vi "MFC_LED_training.vi"() -> ()   [LabVIEW 2021]
uses:
  OdorSensorArray/labview 2016 code/osa_global_save2.vi
  <vilib>/measure/NI_MABase.lvlib
panel:
  in  "Max Voltage 3":dbl=4.5 min=0.0 max=5.0 step=0.1 format="%.2f"
  in  "Min Voltage 3":dbl=0.5 min=0.0 max=5.0 step=0.1 format="%.2f"
  in  "Frequency (Hz) burst":dbl=1.0 step=0.1 format="%.3f"
  in  "Phase_delay":dbl=1.0 step=0.1 format="%.3f"
  in  "Duty cycle (%) 2":dbl=1.0 step=0.1 format="%.3f"
  in  "Function 2":u16(ring) items=["Sine Wave", "Triangle Wave", "Square Wave", "Sawtooth Wave"]
  out "Waveform Chart 2":dbl(graph)
  in  "Duty cycle (%)":dbl=1.0 step=0.1 format="%.3f"
  out "Error U3-2 A0":string
  out "PID / flow":cluster{"Value Read":dbl, "Value Read":dbl}(graph)
  in  "Dilusion_lj2_DAC1":dbl step=0.1 format="%.4f"
  out "Error  PID_Save":string
  out "error write":errorcluster
  in  "Save file":bool
  in  "save data folder":path
  out "appended path":path
  out "AIN0: PID":dbl format="%.6f"
  out "MFC I/O":cluster{"Value Read":dbl, "Value Read":dbl}(graph)
  out "AIN2: MFCr":dbl format="%.6f"
  out "AIN1: MFCw":dbl format="%.6f"
  out "Waveform Chart":dbl(graph)
  out "Error DAC1,B":string
  out "error read":errorcluster
  in  "Background_DAC1":dbl step=0.1 format="%.4f"
  in  "Update Interval (ms)":u32=20
  out "Error_DAC0":string
  in  "Function":u16(ring) items=["Sine Wave", "Triangle Wave", "Square Wave", "Sawtooth Wave"]
  in  "Min Voltage":dbl=0.5 min=0.0 max=5.0 step=0.1 format="%.2f"
  in  "Max Voltage":dbl=4.5 min=0.0 max=5.0 step=0.1 format="%.2f"
  in  "Frequency (Hz)":dbl=1.0 step=0.1 format="%.3f"
  in  "Stop":bool
  # "Updates DAC0 at the specified update interval in order to build time series waveforms.  The\nupdate interval is set to 20 ms by default, but can be set lower based on the execution times\ndiscussed in Section 3.1 of the U3 User's Guide.  Uses the first found U3.\n\nWith a software timed application such as this, you might be able to reduce timing jitter (caused\nby the operating system) by increasing the priority of this process (labview.exe) in Windows\nTask Manager."
  # "MFC"
  # "LED"
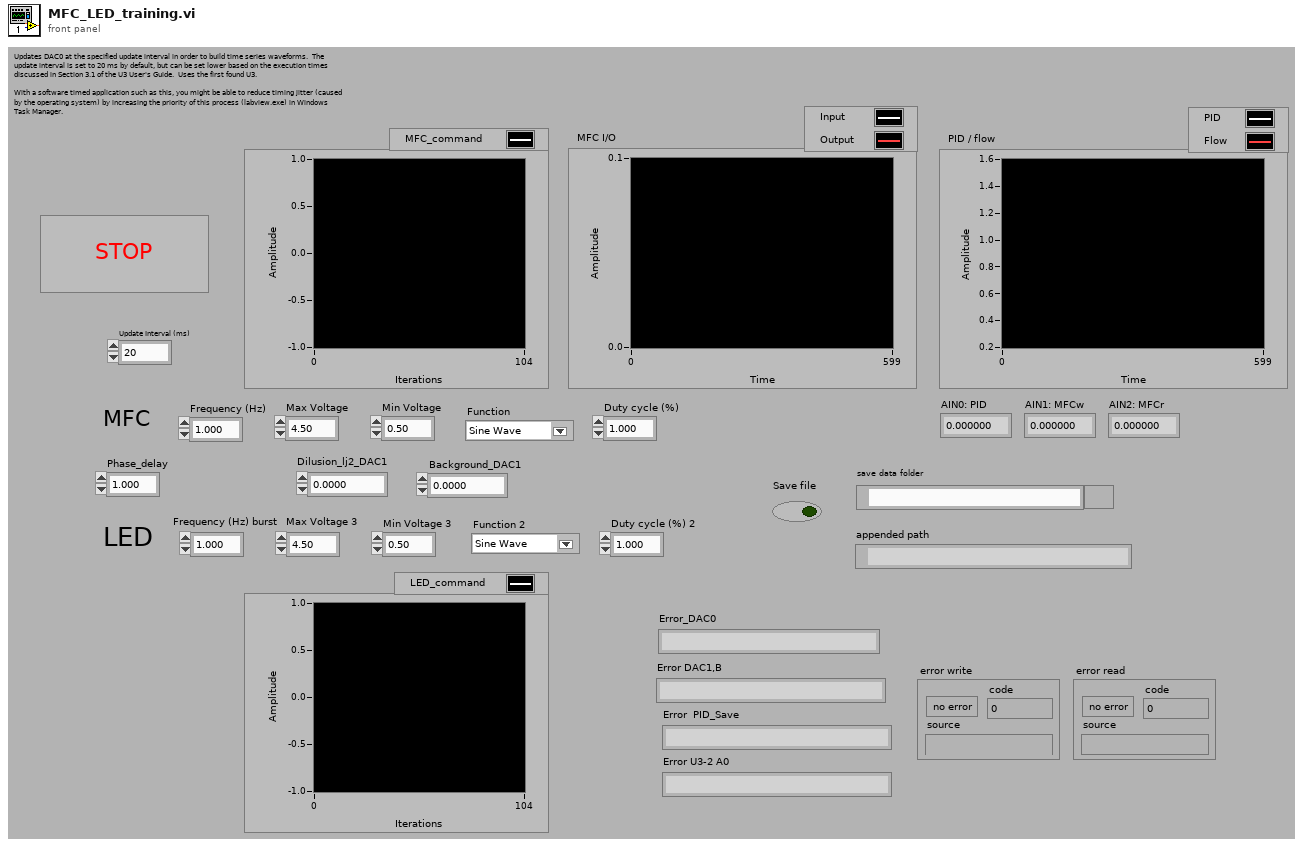
[diagram p1: front panel]
types:
  T1 = enum16{"open", "replace", "create", "open or create", "replace or create", "replace or create with confirmation"}
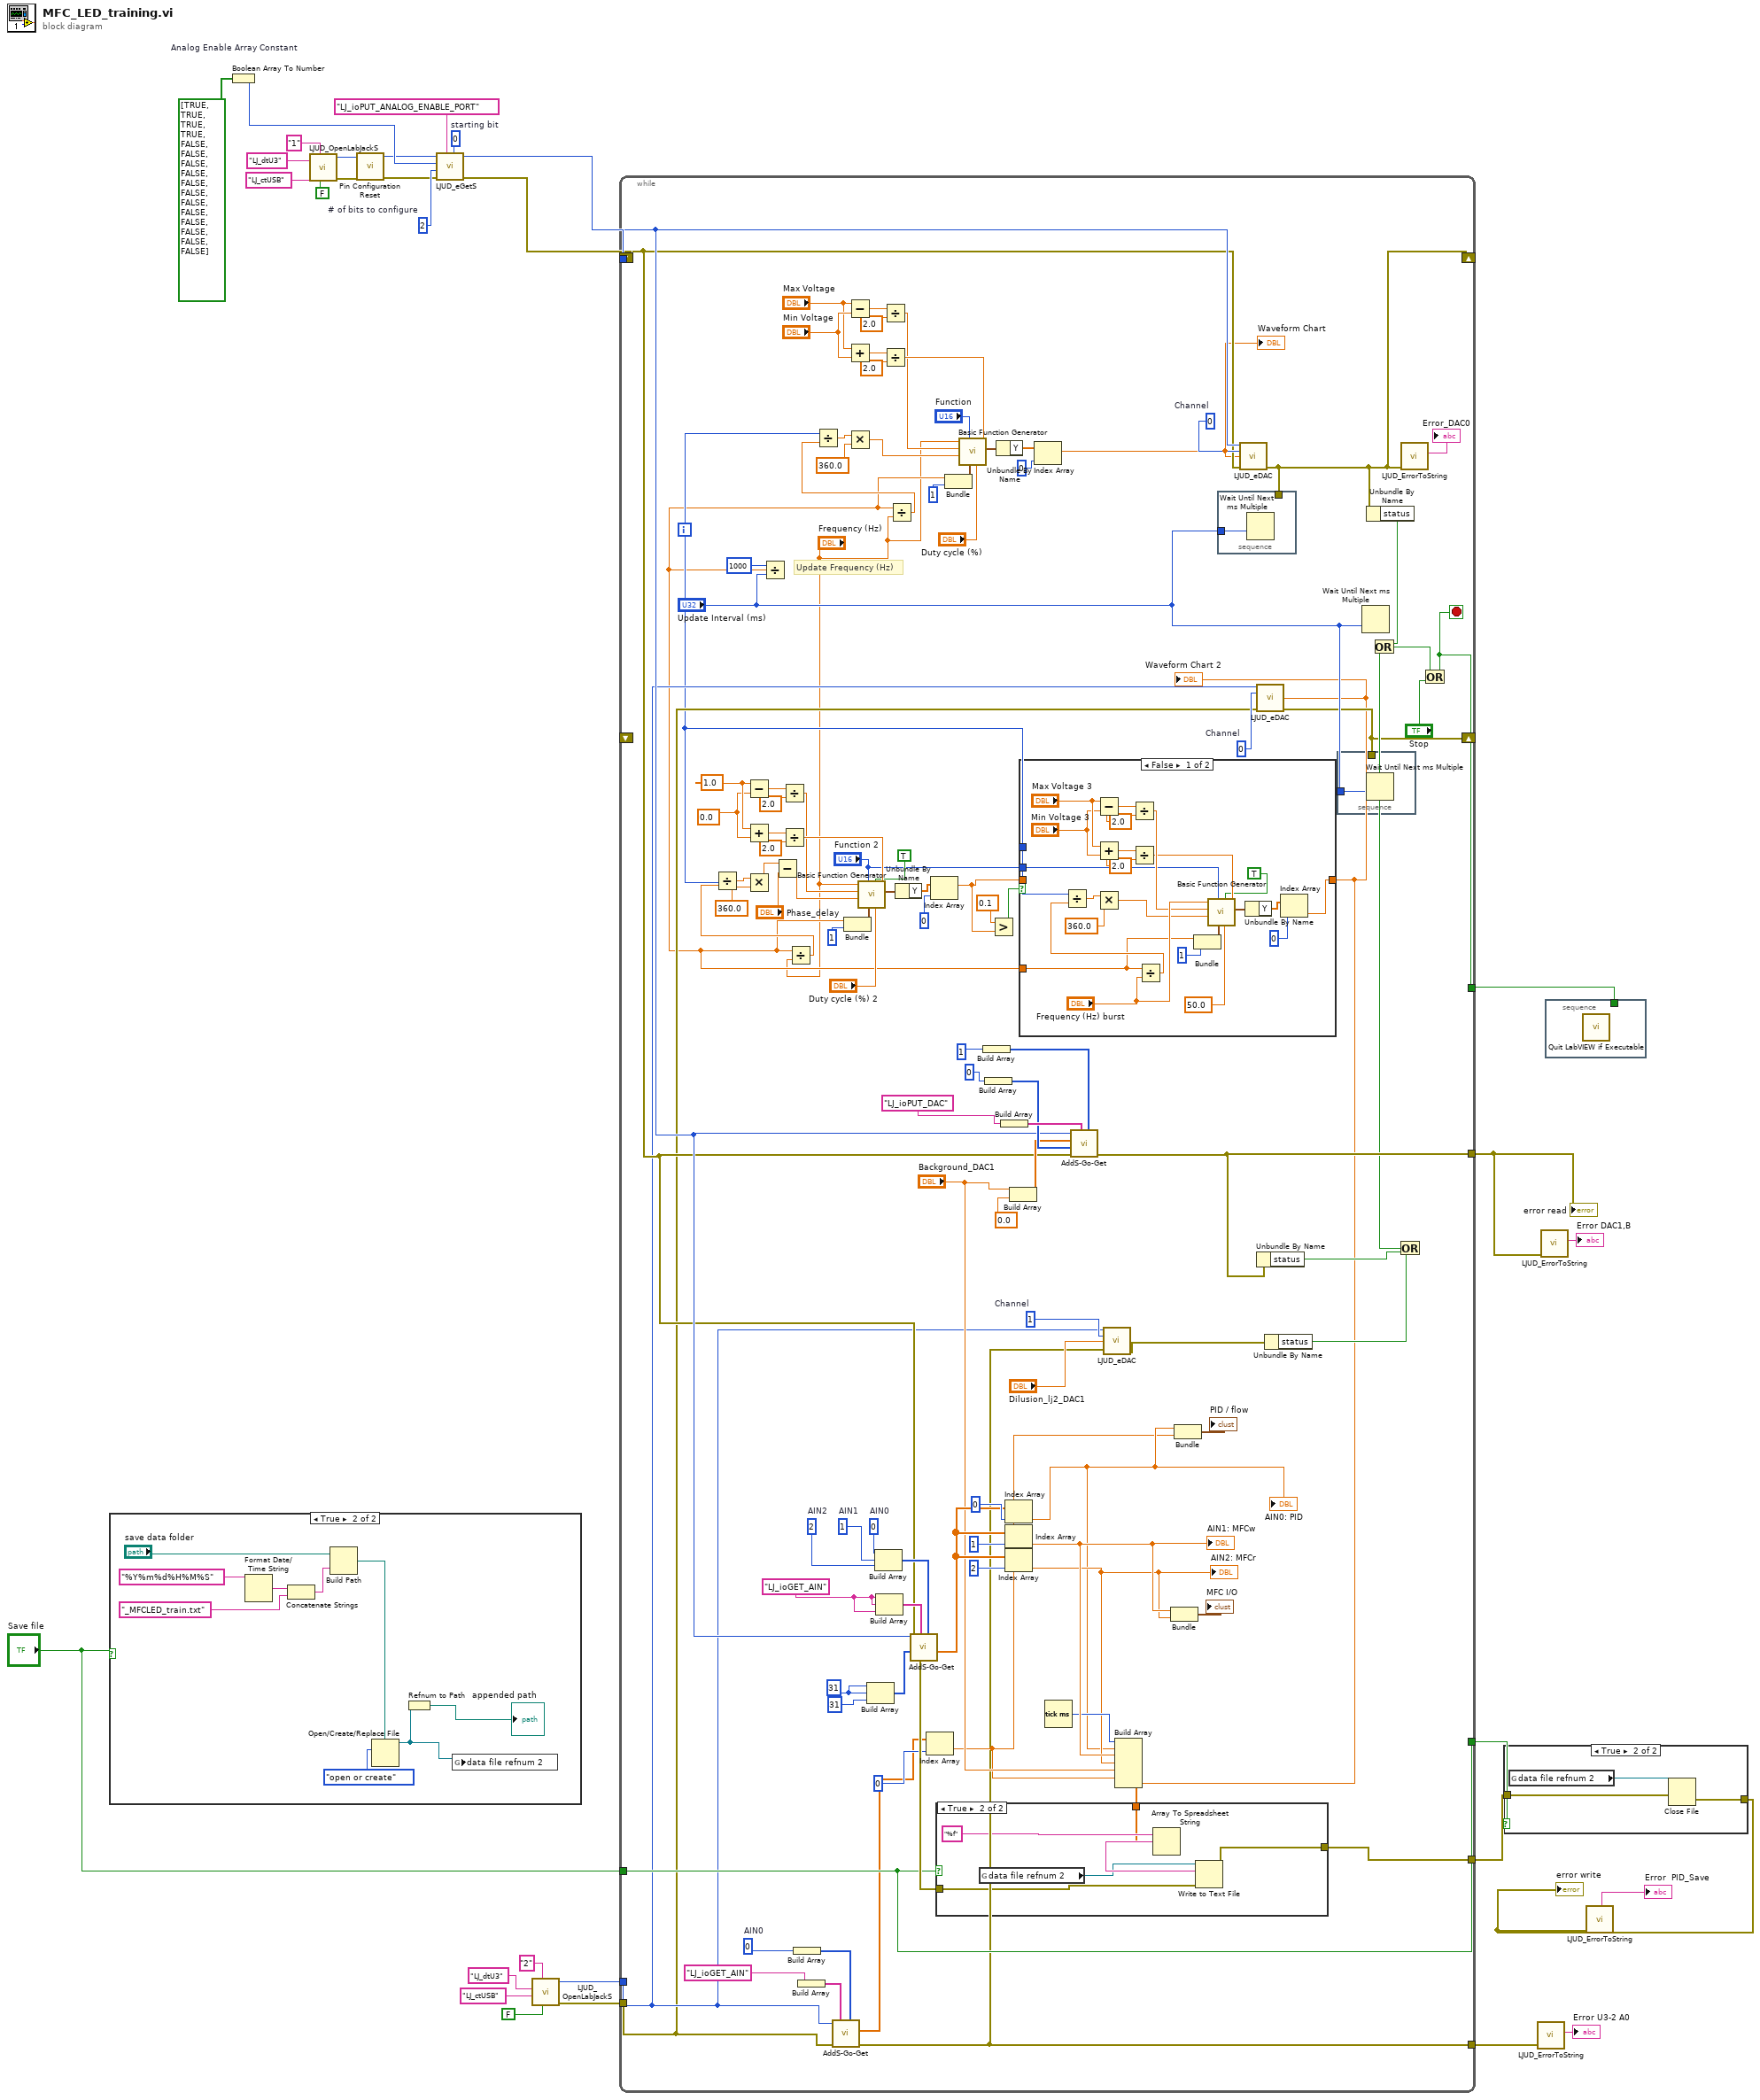
[diagram p0: block diagram]
diagram:
  w19 = 2  # # of bits to configure
  w21 = 0  # starting bit
  w22 = bool[] [TRUE, TRUE, TRUE, TRUE, FALSE, FALSE, FALSE, FALSE, FALSE, FALSE, FALSE, FALSE, FALSE, FALSE, FALSE, FALSE]  # Analog Enable Array Constant
  n1 = case shown="True" "Save file" {
    frame False {
    }
    frame True {
      n2 = Format Date/Time String(time format string (%c)="%Y%m%d%H%M%S") -> (date/time string=w37:string)  [unwired: 2 in]
      n3 = Concatenate Strings(w37, "_MFCLED_train.txt") -> (w39:string)
      n4 = Build Path(base path="save data folder", name or relative path=w39) -> (appended path=w33:path)
      n5 = Open/Create/Replace File(file path (use dialog)=w33, operation (0:open)=T1."open or create") -> (refnum out=w32:refnum<file>)  [unwired: 4 in, 2 out]
      n6 = Refnum to Path(1:w32) -> (0:→"appended path":path)
      n7 = global write "osa_global_save2.vi" "data file refnum 2"(w32) -> ()
    }
  }
  n8 = Boolean Array To Number(Boolean array=w22) -> (number=w18:u32)
  n9 = call "LJUD_OpenLabJackS.vi"("FirstFound"=FALSE, "Address"="1" ("DeviceType"), "ConnectionType"="LJ_ctUSB", "DeviceType"="LJ_dtU3") -> ("error out"=w23:errorcluster, "Handle"=w24:i32)  [unwired: 5 in, 1 out]
  n10 = call "Pin Configuration Reset.vi"("error in"=w23, "Handle In"=w24) -> ("error out"=w16:errorcluster, "Handle Out"=w17:i32)  [unwired: 8 in]
  n11 = call "LJUD_eGetS.vi"("Channel"=w21, "IOType"="LJ_ioPUT_ANALOG_ENABLE_PORT", "error in"=w16, "x1"=w19, "Value Write"=w18, "Handle In"=w17) -> ("error out"=w14:errorcluster, "Handle Out"=w15:i32)  [unwired: 3 in, 1 out]
  n12 = call "LJUD_OpenLabJackS.vi"("FirstFound"=FALSE, "Address"="2", "ConnectionType"="LJ_ctUSB", "DeviceType"="LJ_dtU3") -> ("error out"=w3:errorcluster, "Handle"=w4:i32)  [unwired: 5 in, 1 out]
  n13 = while {
    tunnel: w15 -> [w116]
    shift-left: w14 -> [w115]
    shift-right: [w148] -> _
    tunnel: [w136] -> w31
    tunnel: [w139] -> w29
    tunnel: [w112] -> w13
    tunnel: "Save file" -> [w110]
    tunnel: [w110] -> w11
    tunnel: w4 -> [w73]
    tunnel: w3 -> [w72]
    tunnel: [w95] -> w1
    shift-right: [w57] -> _
    shift-left: _ -> [_]
    i -> [w47]
    stop <- w136 stop-if-true
    w44 = 0.0 ("y")
    w45 = 1.0 ("y")
    w74 = 0  # Channel
    w94 = 1  # Channel
    w106 = 0  # AIN0
    w122 = 2  # AIN2
    w118 = 31 ("AIN0")
    w127 = 1  # AIN1
    w126 = 0  # AIN0
    w119 = "LJ_ioGET_AIN" ("IOType")
    w149 = 0  # Channel
    # "Update Frequency (Hz)"
    n14 = Subtract(x=w45, y=w44) -> (x-y=w69:dbl)
    n15 = Add(x=w45, y=w44) -> (x+y=w66:dbl)
    n16 = Divide(x=u32 1000, y="Update Interval (ms)") -> (x/y=w46:dbl)
    n17 = Divide(x=w69, y=2.0) -> (x/y=w64:dbl)
    n18 = Divide(x=w66, y=2.0) -> (x/y=w65:dbl)
    n19 = Divide(x=w46, y="Frequency (Hz)") -> (x/y=w71:dbl)
    n20 = Divide(x=w47, y=w71) -> (x/y=w70:dbl)
    n21 = Multiply(x=w70, y=360.0) -> (x*y=w55:dbl)
    n22 = Subtract(x=w55, y="Phase_delay") -> (x-y=w54:dbl)
    n23 = Build Array(w106) -> (w107:i32[])
    n24 = Build Array("LJ_ioGET_AIN" ("IOType")) -> (w105:string[])
    n25 = call "AddS-Go-Get.vi"("Channels"=w107, "IOTypes"=w105, "error in"=w72, "Handle In"=w73) -> ("error out"=w95:errorcluster, "Values Read"=w100:dbl[])  [unwired: 5 in, 1 out]
    n26 = Bundle(w46, 1) -> (w61:cluster{dbl, i32})  [unwired: 1 in]
    n27 = Subtract(x="Max Voltage", y="Min Voltage") -> (x-y=w91:dbl)
    n28 = Add(x="Max Voltage", y="Min Voltage") -> (x+y=w88:dbl)
    n29 = call <vilib>:"Basic Function Generator.vi"("offset"=w65, "square wave duty cycle (%)"="Duty cycle (%) 2", "reset signal"=TRUE, "sampling info"=w61, "signal type"="Function 2", "phase"=w54, "amplitude"=w64, "frequency"="Frequency (Hz)") -> ("signal out"=w60:waveform(dbl))  [unwired: 1 in, 2 out]
    n30 = Build Array(w118, w118, 31 ("AIN1")) -> (w123:i32[])
    n31 = Build Array(w126, w127, w122) -> (w130:i32[])
    n32 = Build Array(w119, w119, w119) -> (w131:string[])
    n33 = Divide(x=w91, y=2.0) -> (x/y=w83:dbl)
    n34 = Divide(x=w88, y=2.0) -> (x/y=w84:dbl)
    n35 = Divide(x=w46, y="Frequency (Hz)") -> (x/y=w93:dbl)
    n36 = Divide(x=w47, y=w93) -> (x/y=w92:dbl)
    n37 = Multiply(x=w92, y=360.0) -> (x*y=w81:dbl)
    n38 = Unbundle By Name(w60) -> ("Y"=w51:dbl[])
    n39 = call "AddS-Go-Get.vi"("Channels"=w130, "IOTypes"=w131, "error in"=w115, "x1"=w123, "Handle In"=w116) -> ("error out"=w113:errorcluster, "Values Read"=w111:dbl[])  [unwired: 4 in, 1 out]
    n40 = Index Array(array=w100, index=0 ("Index")) -> (element=w99:dbl)
    n41 = Index Array(array=w51, index=0 ("Index")) -> (element=w48:dbl)
    n42 = Bundle(w46, 1) -> (w79:cluster{dbl, i32})  [unwired: 1 in]
    n43 = call <vilib>:"Basic Function Generator.vi"("offset"=w84, "square wave duty cycle (%)"="Duty cycle (%)", "sampling info"=w79, "signal type"="Function", "phase"=w81, "amplitude"=w83, "frequency"="Frequency (Hz)") -> ("signal out"=w78:waveform(dbl))  [unwired: 2 in, 2 out]
    n44 = Build Array(1) -> (w145:i32[])
    n45 = Build Array(0) -> (w140:i32[])
    n46 = Greater?(x=0.1 ("y"), y=w48) -> (0:w49:bool)
    n47 = Unbundle By Name(w78) -> ("Y"=w77:dbl[])
    n48 = Build Array("LJ_ioPUT_DAC" ("IOType")) -> (w146:string[])
    n49 = Index Array(array=w111, index=0 ("Index")) -> (element=w102:dbl)
    "AIN0: PID" <- w102
    n50 = Index Array(array=w111, index=1 ("Index")) -> (element=w120:dbl)
    "AIN1: MFCw" <- w120
    n51 = Index Array(array=w111, index=2 ("Index")) -> (element=w114:dbl)
    "AIN2: MFCr" <- w114
    n52 = Build Array("Background_DAC1", 0.0 ("Input Element")) -> (w135:dbl[])
    n53 = case shown="False" w49 {
      tunnel: [w157 w176] -> w41
      tunnel: w48 -> [_ w176]
      tunnel: w47 -> [w156 _]
      tunnel: w46 -> [w155 _]
      tunnel: "Function 2" -> [w153 _]
      frame False {
        n54 = Subtract(x="Max Voltage 3", y="Min Voltage 3") -> (x-y=w166:dbl)
        n55 = Add(x="Max Voltage 3", y="Min Voltage 3") -> (x+y=w167:dbl)
        n56 = Divide(x=w166, y=2.0) -> (x/y=w171:dbl)
        n57 = Divide(x=w167, y=2.0) -> (x/y=w170:dbl)
        n58 = Divide(x=w155, y="Frequency (Hz) burst") -> (x/y=w164:dbl)
        n59 = Divide(x=w156, y=w164) -> (x/y=w165:dbl)
        n60 = Multiply(x=w165, y=360.0) -> (x*y=w152:dbl)
        n61 = Bundle(w155, 1) -> (w173:cluster{dbl, i32})  [unwired: 1 in]
        n62 = call <vilib>:"Basic Function Generator.vi"("offset"=w170, "square wave duty cycle (%)"=50.0 ("y"), "reset signal"=TRUE, "sampling info"=w173, "signal type"=w153, "phase"=w152, "amplitude"=w171, "frequency"="Frequency (Hz) burst") -> ("signal out"=w174:waveform(dbl))  [unwired: 1 in, 2 out]
        n63 = Unbundle By Name(w174) -> ("Y"=w175:dbl[])
        n64 = Index Array(array=w175, index=0 ("Index")) -> (element=w157:dbl)
      }
      frame True {
      }
    }
    "Waveform Chart 2" <- w41
    n65 = Index Array(array=w77, index=0 ("Index")) -> (element=w98:dbl)
    "Waveform Chart" <- w98
    n66 = Tick Count (ms)() -> (millisecond timer value=w117:u32)
    n67 = call "AddS-Go-Get.vi"("Channels"=w145, "IOTypes"=w146, "error in"=w115, "x1"=w140, "Values Write"=w135, "Handle In"=w116) -> ("error out"=w139:errorcluster)  [unwired: 3 in, 2 out]
    n68 = call "LJUD_eDAC.vi"("Handle In"=w73, "Channel"=w94, "Voltage"="Dilusion_lj2_DAC1", "error in"=w95) -> ("error out"=w96:errorcluster)  [unwired: 10 in, 1 out]
    n69 = Build Array(w117, w102, w120, w114, "Background_DAC1", w99, w41) -> (w109:dbl[])
    n70 = case shown="True" w110 {
      tunnel: w113 -> [w178 w183]
      tunnel: [w178 w182] -> w112
      tunnel: w109 -> [_ w179]
      frame False {
      }
      frame True {
        n71 = global read "osa_global_save2.vi" "data file refnum 2"() -> (w180:refnum<file>)
        n72 = Array To Spreadsheet String(array=w179, 3:"%f") -> (spreadsheet string=w181:string)  [unwired: 1 in]
        n73 = Write to Text File(file (use dialog)=w180, text=w181, error in=w183) -> (error out=w182:errorcluster)  [unwired: 1 in, 2 out]
      }
    }
    n74 = Bundle("Value Read"=w120, "Value Read"=w114) -> (→"MFC I/O":cluster{"Value Read":dbl, "Value Read":dbl})  [unwired: 1 in]
    n75 = Bundle("Value Read"=w102, "Value Read"=w99) -> (→"PID / flow":cluster{"Value Read":dbl, "Value Read":dbl})  [unwired: 1 in]
    n76 = call "LJUD_eDAC.vi"("Handle In"=w116, "Channel"=w149, "Voltage"=w98, "error in"=w115) -> ("error out"=w148:errorcluster)  [unwired: 10 in, 1 out]
    n77 = stacked-sequence {
      tunnel: "Update Interval (ms)" -> [w185]
      tunnel: w148 -> [_]
      frame #0 {
        n78 = Wait Until Next ms Multiple(millisecond multiple=w185) -> ()  [unwired: 1 out]
      }
    }
    n79 = call "LJUD_eDAC.vi"("Handle In"=w73, "Channel"=w74, "Voltage"=w41, "error in"=w72) -> ("error out"=w57:errorcluster)  [unwired: 10 in, 1 out]
    n80 = Unbundle By Name(w139) -> ("status"=w132:bool)
    n81 = Unbundle By Name(w96) -> ("status"=w133:bool)
    n82 = stacked-sequence {
      tunnel: "Update Interval (ms)" -> [w177]
      tunnel: w57 -> [_]
      frame #0 {
        n83 = Wait Until Next ms Multiple(millisecond multiple=w177) -> ()  [unwired: 1 out]
      }
    }
    n84 = Wait Until Next ms Multiple(millisecond multiple="Update Interval (ms)") -> ()  [unwired: 1 out]
    n85 = Unbundle By Name(w148) -> ("status"=w138:bool)
    n86 = Or(x=w133, y=w132) -> (x .or. y?=w134:bool)
    n87 = Or(x=w138, y=w134) -> (x .or. y?=w137:bool)
    n88 = call "LJUD_ErrorToString.vi"("error in"=w148) -> ("String"=→"Error_DAC0":string)  [unwired: 10 in]
    n89 = Or(x=w137, y="Stop") -> (x .or. y?=w136:bool)
  }
  "error read" <- w29
  n90 = case shown="True" w11 {
    tunnel: w13 -> [w186 w189]
    tunnel: [w186 w188] -> w9
    frame False {
    }
    frame True {
      n91 = global read "osa_global_save2.vi" "data file refnum 2"() -> (w187:refnum<file>)
      n92 = Close File(refnum=w187, error in=w189) -> (error out=w188:errorcluster)  [unwired: 1 out]
    }
  }
  "error write" <- w9
  n93 = call "LJUD_ErrorToString.vi"("error in"=w1) -> ("String"=→"Error U3-2 A0":string)  [unwired: 10 in]
  n94 = call "LJUD_ErrorToString.vi"("error in"=w29) -> ("String"=→"Error DAC1,B":string)  [unwired: 10 in]
  n95 = stacked-sequence {
    tunnel: w31 -> [_]
    frame #0 {
      n96 = call "Quit LabVIEW if Executable.vi"() -> ()  [unwired: 1 in]
    }
  }
  n97 = call "LJUD_ErrorToString.vi"("error in"=w9) -> ("String"=→"Error  PID_Save":string)  [unwired: 10 in]
